vi "Get Control Values.vi"(6 "class names":string[](array[string]), 8 "error in":errorcluster, 11 "refnums in":refnum<vi>[](array[refnum])) -> (0 "error out":errorcluster, 2 "values":dbl[](array[numeric]), 3 "refnums out":refnum<vi>[](array[refnum]))   [LabVIEW 2020]
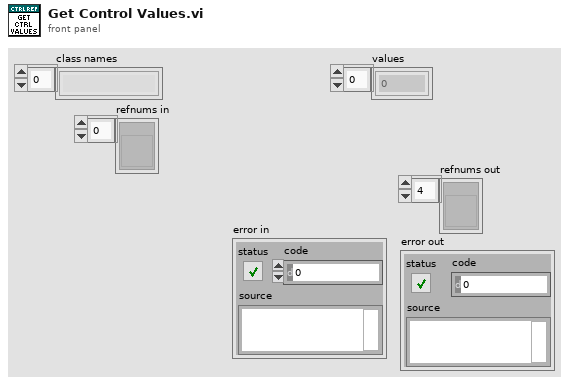
[diagram p1: front panel]
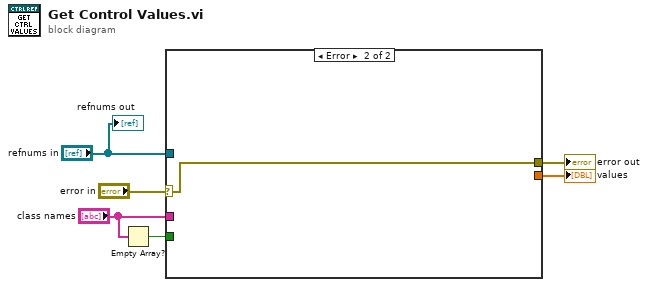
[diagram p0: block diagram]
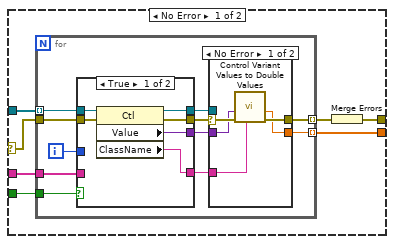
[diagram p2: hidden frame]
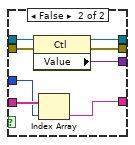
[diagram p3: hidden frame]
diagram:
  n1 = Empty Array?(array="class names") -> (empty?=w2:bool)
  n2 = case shown="Error" "error in" {
    selector: "error in" -> [w10 w45]
    tunnel: "refnums in" -> [w12 _]
    tunnel: [w11 w45] -> w5
    tunnel: [w9 _] -> w3
    tunnel: w2 -> [w8 _]
    tunnel: "class names" -> [w7 _]
    frame No Error {
      n3 = for {
        tunnel: w12 -> [w24] mode=indexing
        tunnel: [w22] -> w13 mode=indexing
        tunnel: [w20] -> w9 mode=indexing
        tunnel: w10 -> [w19]
        tunnel: w8 -> [w18]
        tunnel: w7 -> [w15]
        i -> [w14]
        n4 = case shown="True" w18 {
          tunnel: w24 -> [w30 w38]
          tunnel: [w29 w37] -> w23
          tunnel: [w28 w36] -> w21
          tunnel: w19 -> [w27 w35]
          tunnel: [w26 w34] -> w17
          tunnel: [w25 w32] -> w16
          tunnel: w15 -> [_ w33]
          tunnel: w14 -> [_ w31]
          frame True {
            n5 = property class="Ctl"(reference=w30, error in=w27) -> (reference out=w29:refnum<vi>, error out=w28:errorcluster, "Value"=w26:variant, "ClassName"=w25:string)
          }
          frame False {
            n6 = property class="Ctl"(reference=w38, error in=w35) -> (reference out=w37:refnum<vi>, error out=w36:errorcluster, "Value"=w34:variant)
            n7 = Index Array(array=w33, index=w31) -> (element=w32:string)
          }
        }
        n8 = case shown="No Error" w21 {
          selector: w21 -> [w43 w44]
          tunnel: w23 -> [_ _]
          tunnel: [w42 w44] -> w22
          tunnel: [w39 _] -> w20
          tunnel: w17 -> [w40 _]
          tunnel: w16 -> [w41 _]
          frame No Error {
            n9 = call "Control Variant Values to Double Values.vi"("class names"=w41, "error in (no error)"=w43, "variant values"=w40) -> ("error out"=w42:errorcluster, "values"=w39:dbl)  [unwired: 7 in]
          }
          frame Error {
          }
        }
      }
      n10 = Merge Errors(w13) -> (w11:errorcluster)
    }
    frame Error {
    }
  }
  "error out" <- w5
  "values" <- w3
  "refnums out" <- "refnums in"
